vi "Throttle Percent To Value.vi"(11 "throttle percent":dbl) -> (2 "throttle percent (actual)":dbl, 3 "throttle value":u16)   [LabVIEW 2023, in "Aurora64b66b Utilities Host.lvlib"]
uses:
  Aurora64b66b Utilities Host.lvlib
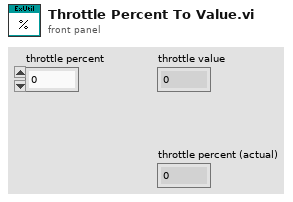
[diagram p1: front panel]
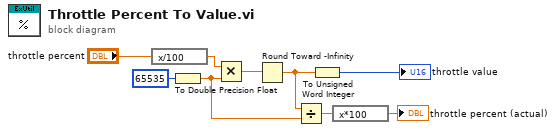
[diagram p0: block diagram]
diagram:
  n1 = expression code="x/100"("throttle percent") -> (w5:dbl)
  n2 = To Double Precision Float(number=65535) -> (double precision float=w3:dbl)
  n3 = Multiply(x=w5, y=w3) -> (x*y=w7:dbl)
  n4 = Round Toward -Infinity(1:w7) -> (0:w4:dbl)
  n5 = Divide(x=w4, y=w3) -> (x/y=w2:dbl)
  n6 = To Unsigned Word Integer(number=w4) -> (unsigned 16bit integer=→"throttle value":u16)
  n7 = expression code="x*100"(w2) -> (→"throttle percent (actual)":dbl)
